vi "test-trapezoid-profile-cont-under-vel-change.vi"() -> (3 "Test Passed":bool)   [LabVIEW 2019]
uses:
  <vilib>/Rock Robotics/WPI/ThirdParty/JAS_Junk/TrajLib/TRAPEZOID_PROFILE_STATE.ctl
  <vilib>/Rock Robotics/WPI/ThirdParty/JAS_Junk/TrajLib/TRAPEZOID_PROFILE.ctl
  <vilib>/Rock Robotics/WPI/ThirdParty/JAS_Junk/TrajLib/TRAPEZOID_PROFILE_CONSTRAINT.ctl
  <vilib>/Rock Robotics/WPI/ThirdParty/JAS_Junk/TrajLib/TrapProfile_Direct.vi
  <vilib>/Rock Robotics/WPI/ThirdParty/JAS_Junk/TrajLib/TrapProfile_ShouldFlipAcceleration.vi
  <vilib>/Rock Robotics/SystemInterfaces/NetworkCommunication/NetComm_UsageReport_report.vi
  <vilib>/Rock Robotics/WPI/ThirdParty/JAS_Junk/TrajLib/Util_LibraryGlobals.vi
  <vilib>/Rock Robotics/WPI/ThirdParty/JAS_Junk/TrajLib/Trajectory_Library.lvlib
panel:
  out "ApproxEquals 2":bool
  out "ApproxEquals":bool
  out "Equal":bool
  out "TRAPEZOID_PROFILE":T1 {"Goal"."Velocity" format="%16_6e"; "Goal"."Position" format="%16_6e"; "Initial"."Velocity" format="%16_6e"; "Initial"."Position" format="%16_6e"; "Constraints"."MaxAcceleration" format="%16_6e"; "Constraints"."MaxVelocity" format="%16_6e"; "EndDecel" format="%16_6e"; "EndFullSpeed" format="%16_6e"; "EndAccel" format="%16_6e"}
  out "State":T3 {"Velocity" format="%16_6e"; "Position" format="%16_6e"}
  out "Waveform Chart":T4(graph)
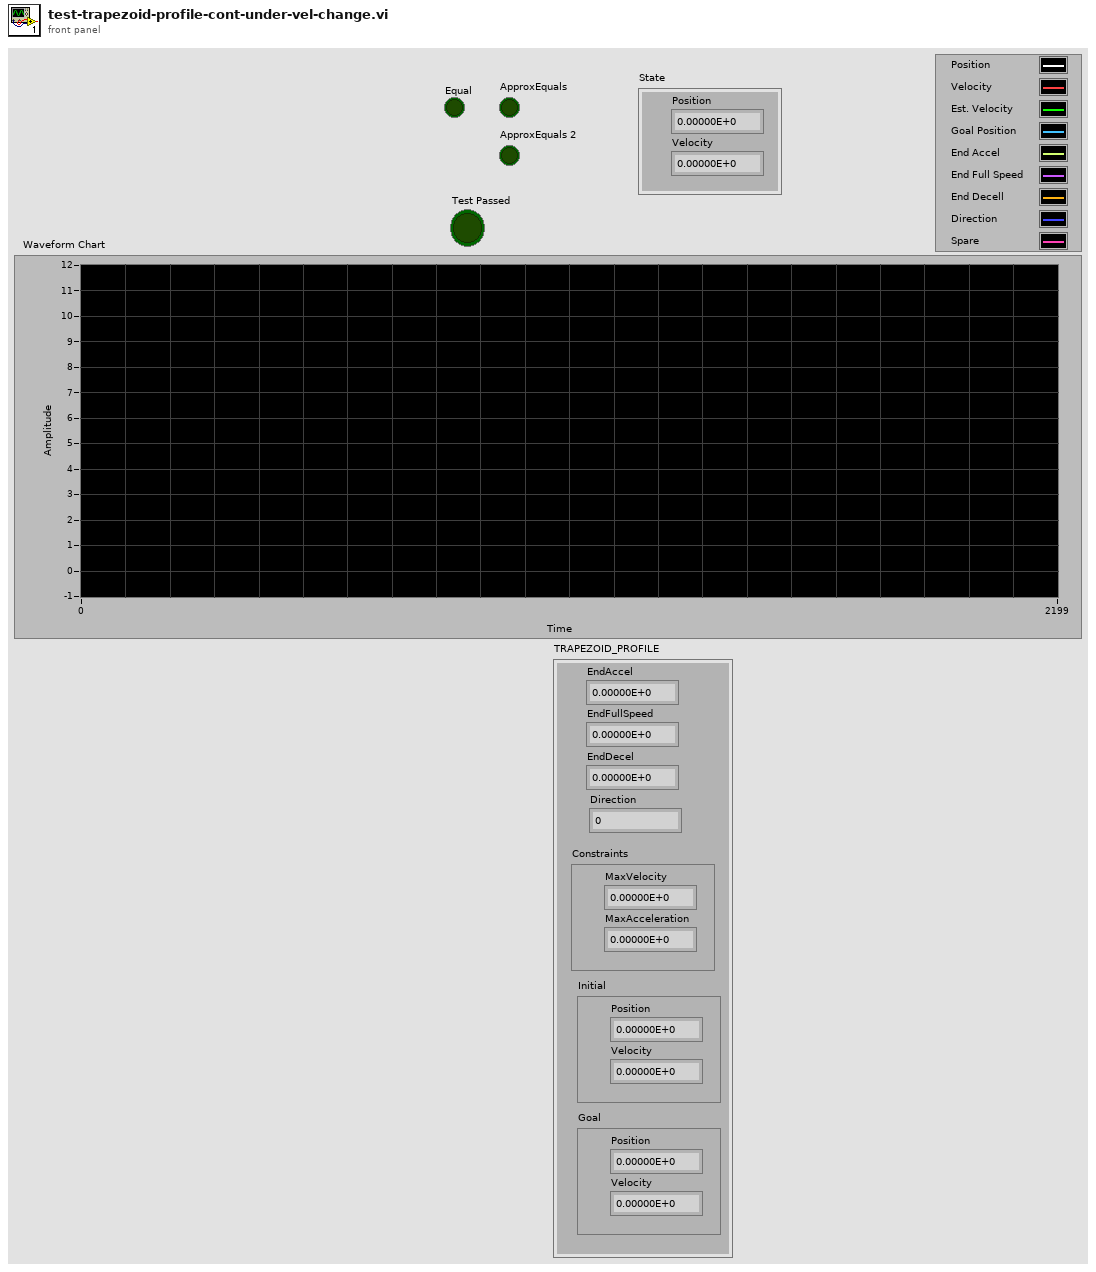
[diagram p1: front panel]
types:
  T1 = typedef "Trajectory_Library.lvlib/TRAPEZOID_PROFILE.ctl" = cluster{"EndAccel":dbl, "EndFullSpeed":dbl, "EndDecel":dbl, "Direction":i32, "Constraints":T2, "Initial":T3, "Goal":T3}
  T2 = typedef "Trajectory_Library.lvlib/TRAPEZOID_PROFILE_CONSTRAINT.ctl" = cluster{"MaxVelocity":dbl, "MaxAcceleration":dbl}
  T3 = typedef "Trajectory_Library.lvlib/TRAPEZOID_PROFILE_STATE.ctl" = cluster{"Position":dbl, "Velocity":dbl}
  T4 = cluster{"Position":dbl, "Velocity":dbl, dbl, "Position":dbl, "EndAccel":dbl, "EndFullSpeed":dbl, "EndDecel":dbl, "Direction":i32, "Position":dbl}
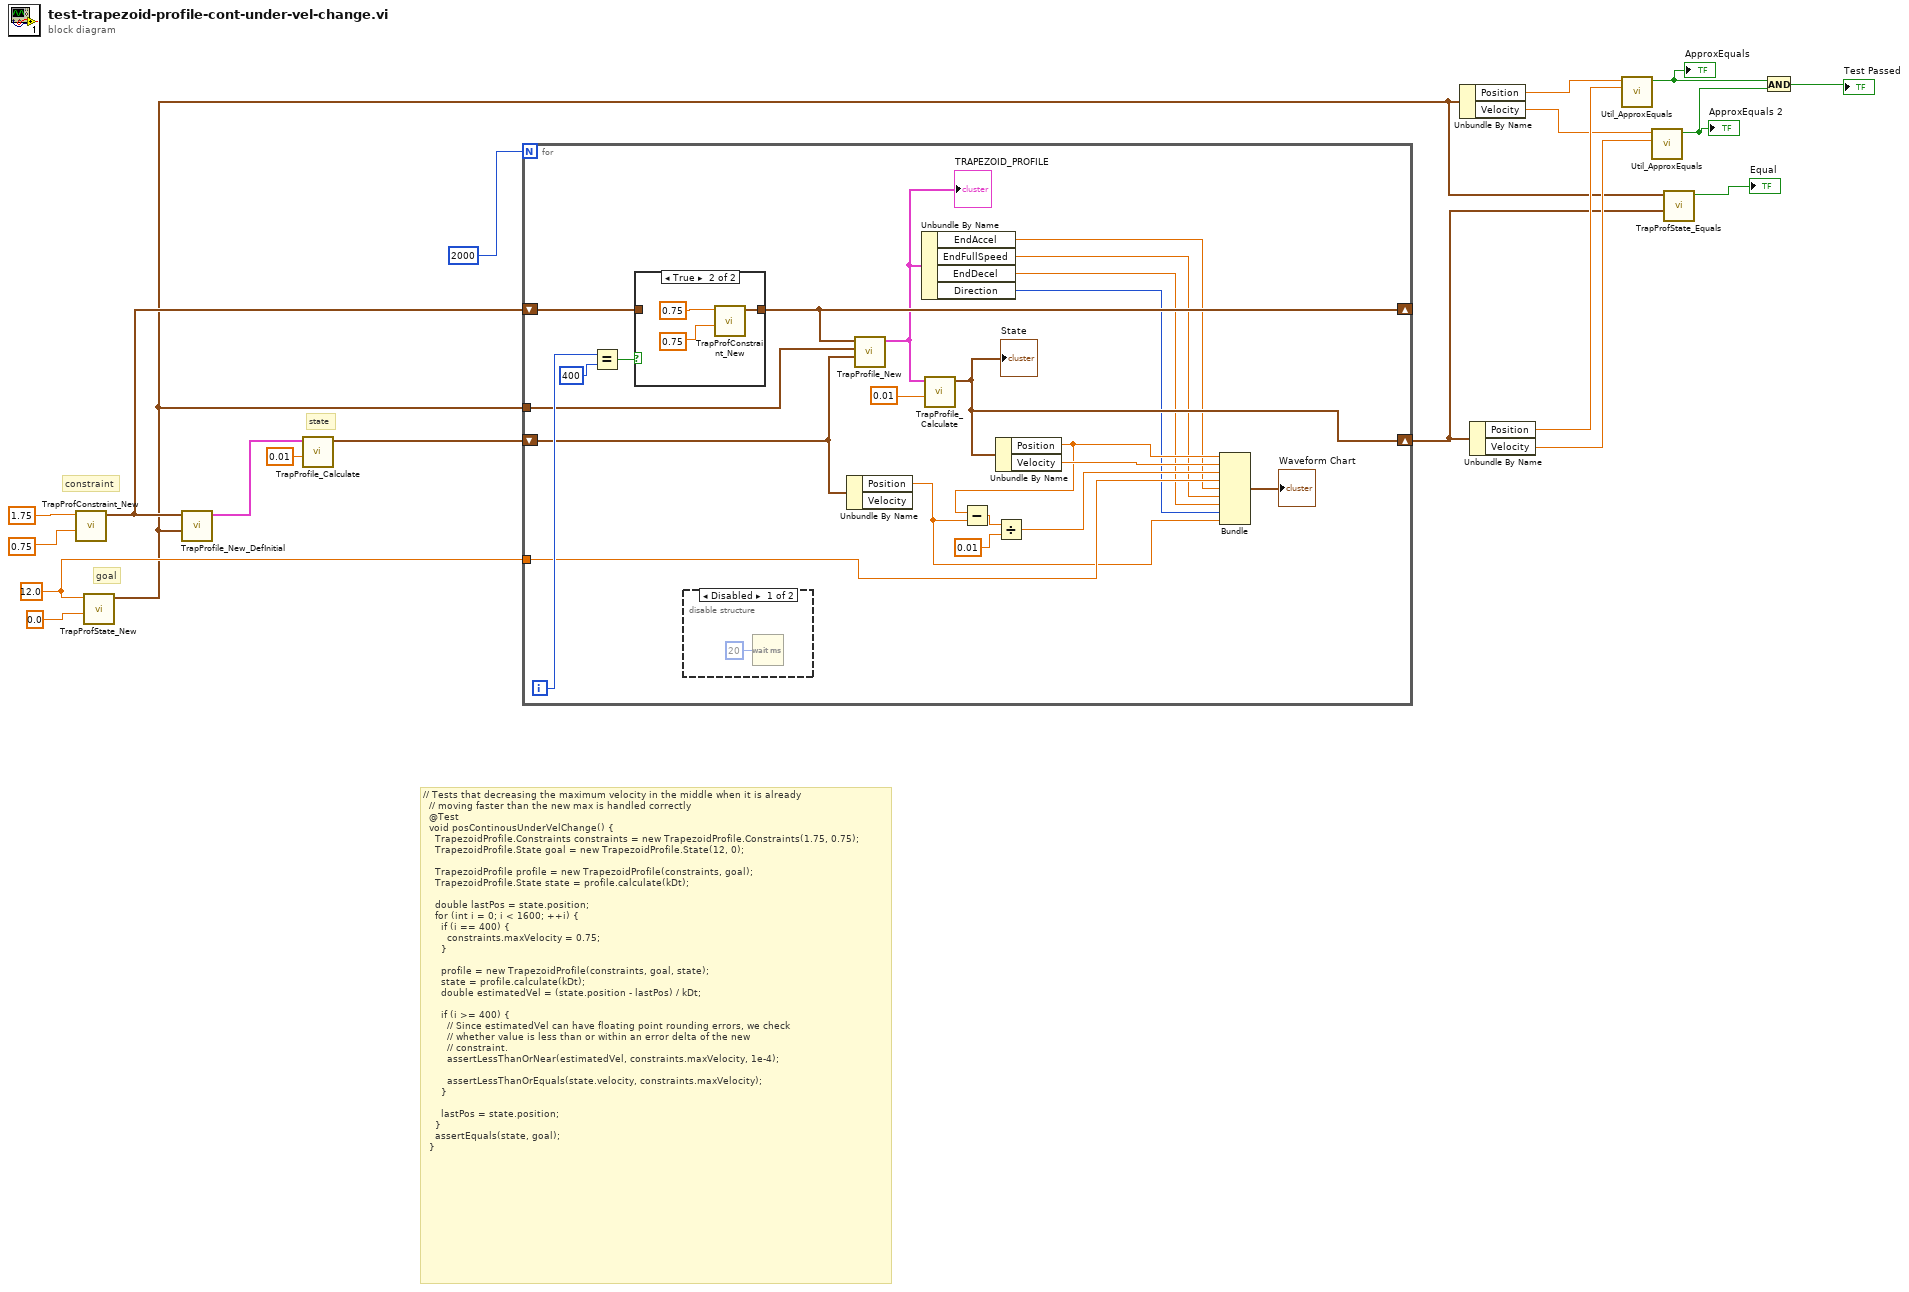
[diagram p0: block diagram]
diagram:
  w11 = 12.0 ("Position")
  # "// Tests that decreasing the maximum velocity in the middle when it is already\n  // moving faster than the new max is handled correctly\n  @Test\n  void posContinousUnderVelChange() {\n    TrapezoidProfile.Constraints constraints = new TrapezoidProfile.Constraints(1.75, 0.75);\n    TrapezoidProfile.State goal = new TrapezoidProfile.State(12, 0);\n\n    TrapezoidProfile profile = new TrapezoidProfile(constraints, goal);\n    TrapezoidProfile.State state = profile.calculate(kDt);\n\n    double lastPos = state.position;\n    for (int i = 0; i < 1600; ++i) {\n      if (i == 400) {\n        constraints.maxVelocity = 0.75;\n      }\n\n      profile = new TrapezoidProfile(constraints, goal, state);\n      state = profile.calculate(kDt);\n      double estimatedVel = (state.position - lastPos) / kDt;\n\n      if (i >= 400) {\n        // Since estimatedVel can have floating point rounding errors, we check\n        // whether value is less than or within an error delta of the new\n        // constraint.\n        assertLessThanOrNear(estimatedVel, constraints.maxVelocity, 1e-4);\n\n        assertLessThanOrEquals(state.velocity, constraints.maxVelocity);\n      }\n\n      lastPos = state.position;\n    }\n    assertEquals(state, goal);\n  }"
  # "goal"
  # "state"
  # "constraint"
  n1 = call <vilib>:"TrapProfConstraint_New.vi"("Max Accel"=0.75, "Max Speed (M/S)"=1.75) -> ("TRAPEZOID_PROFILE_CONSTRAINT"=w12:T2)  [unwired: 9 in]
  n2 = call <vilib>:"TrapProfState_New.vi"("Velocity"=0.0, "Position"=w11) -> ("TRAPEZOID_PROFILE_STATE"=w1:T3)  [unwired: 9 in]
  n3 = call <vilib>:"TrapProfile_New_DefInitial.vi"("Goal"=w1, "Constraints"=w12) -> ("TRAPEZOID_PROFILE"=w15:T1)  [unwired: 9 in]
  n4 = call <vilib>:"TrapProfile_Calculate.vi"("Time"=0.01, "TRAPEZOID_PROFILE"=w15) -> ("State"=w13:T3)  [unwired: 9 in]
  n5 = for {
    N: 2000 -> [_]
    shift-right: [w27] -> w2
    shift-left: w13 -> [w32]
    shift-right: [w35] -> _
    shift-left: w12 -> [w36]
    tunnel: w1 -> [w34]
    tunnel: w11 -> [w26]
    i -> [w38]
    n6 = Equal?(x=w38, y=400) -> (x = y?=w39:bool)
    n7 = case shown="True" w39 {
      tunnel: [w43 w44] -> w35
      tunnel: w36 -> [w43 _]
      frame False {
      }
      frame True {
        n8 = call <vilib>:"TrapProfConstraint_New.vi"("Max Accel"=0.75, "Max Speed (M/S)"=0.75) -> ("TRAPEZOID_PROFILE_CONSTRAINT"=w44:T2)  [unwired: 9 in]
      }
    }
    n9 = disable-structure shown="Disabled" {
      frame Disabled {
        n10 = Wait (ms)(milliseconds to wait=u32 20) -> ()  [unwired: 1 out]
      }
      frame Enabled {
      }
    }
    n11 = Unbundle By Name(w32) -> ("Position"=w20:dbl)  [unwired: 1 out]
    n12 = call <vilib>:"TrapProfile_New.vi"("Initial"=w32, "Goal"=w34, "Constraints"=w35) -> ("TRAPEZOID_PROFILE"=w25:T1)  [unwired: 8 in]
    "TRAPEZOID_PROFILE" <- w25
    n13 = Unbundle By Name(w25) -> ("EndAccel"=w24:dbl, "EndFullSpeed"=w23:dbl, "EndDecel"=w22:dbl, "Direction"=w21:i32)
    n14 = call <vilib>:"TrapProfile_Calculate.vi"("Time"=0.01, "TRAPEZOID_PROFILE"=w25) -> ("State"=w27:T3)  [unwired: 9 in]
    "State" <- w27
    n15 = Unbundle By Name(w27) -> ("Position"=w31:dbl, "Velocity"=w40:dbl)
    n16 = Subtract(x=w31, y=w20) -> (x-y=w30:dbl)
    n17 = Divide(x=w30, y=0.01) -> (x/y=w28:dbl)
    n18 = Bundle("Position"=w31, "Velocity"=w40, w28, "Position"=w26, "EndAccel"=w24, "EndFullSpeed"=w23, "EndDecel"=w22, "Direction"=w21, "Position"=w20) -> (→"Waveform Chart":T4)  [unwired: 1 in]
  }
  n19 = Unbundle By Name(w1) -> ("Position"=w10:dbl, "Velocity"=w8:dbl)
  n20 = Unbundle By Name(w2) -> ("Position"=w9:dbl, "Velocity"=w6:dbl)
  n21 = call <vilib>:"Util_ApproxEquals.vi"("Value 2"=w9, "Value 1"=w10) -> ("ApproxEquals"=w4:bool)  [unwired: 9 in]
  "ApproxEquals" <- w4
  n22 = call <vilib>:"Util_ApproxEquals.vi"("Value 2"=w6, "Value 1"=w8) -> ("ApproxEquals"=w3:bool)  [unwired: 9 in]
  "ApproxEquals 2" <- w3
  n23 = call <vilib>:"TrapProfState_Equals.vi"("TRAPEZOID_PROFILE_STATE 2"=w2, "TRAPEZOID_PROFILE_STATE"=w1) -> ("Equal"=→"Equal":bool)  [unwired: 9 in]
  n24 = And(x=w4, y=w3) -> (x .and. y?=→"Test Passed":bool)
